vi "Defender.vi"(0 "command\nenum":T13, 2 "Our Robot":T5={"id"=0, "function"=enum."Attacker", "x"=0.0, "y"=0.0, "orientation"=0.0, "v_tangent"=0.0, "v_normal"=0.0, "v_ang"=0.0, "kick_x"=0.0, "kick_z"=0.0, "dribble"=FALSE, "Timestamp"=timestamp(0 s since 1904-01-01), "estimatives"={"est_v_tangent"=0.0, "est_v_normal"=0.0, "est_vx"=0.0, "est_vy"=0.0, "Pos Robot Est"=[]}, "dest_x_kick"=0.0, "dest_y_kick"=0.0, "Gap Coord"=[], "States"=enum."GoToTangent", "Path "=[], "Path  Smooth"=[], "Dest"=[]}, 3 "Atacando contra?":bool=TRUE, 4 "Total de n\natacantes":i32, 5 "Enemy Robots":T5={"id"=0, "function"=enum."Attacker", "x"=0.0, "y"=0.0, "orientation"=0.0, "v_tangent"=0.0, "v_normal"=0.0, "v_ang"=0.0, "kick_x"=0.0, "kick_z"=0.0, "dribble"=FALSE, "Timestamp"=timestamp(0 s since 1904-01-01), "estimatives"={"est_v_tangent"=0.0, "est_v_normal"=0.0, "est_vx"=0.0, "est_vy"=0.0, "Pos Robot Est"=[]}, "dest_x_kick"=0.0, "dest_y_kick"=0.0, "Gap Coord"=[], "States"=enum."GoToTangent", "Path "=[], "Path  Smooth"=[], "Dest"=[]}, 6 "Defensores":u32[](array[numeric]), 7 "geometry":T11, 8 "N atacantes":u32[](array[numeric]), 10 "Total de robos":u32[](array[numeric]), 11 "AI Parameters":T3={"GotoKick"={"Dist do cone a frente"=150.0, "attacker farback"=1500.0, "Perto"=300.0, "min dist to kick"=150.0, "kick eps"=0.0, "Time to transition"=0.05}, "Attacker"={"CC chute"=0.09, "CC passe"=0.045, "Kick Force"=100.0, "ball-robot Kick"=200.0, "ball-robot Pass"=0.3, "drible\nAttk"=FALSE}, "Defender"={"D max"=1700.0, "Vel p/ robô av"=1000.0, "Kick Force"=100.0, "D atk-def"=0.0, "D farback"=0.0, "drible\ndef"=FALSE, "drible\ngoalie"=FALSE}, "Timeout"={"Field/v in x"=6.0, "Dist Robots"=300, "Dist up in y"=300}, "Pose Striker"={"dist"=200.0, "Numeric"=-4.0, "dist 2"=200.0, "drible\nstriker"=FALSE}, "Dist Stop"=300.0, "D ball out"=200, "D central gap "=150.0, "T pass"=0.0, "Force ++"=0.0, "range kick"=0.0, "Chute alto"=TRUE, "Marcador novo"=TRUE, "drible"=FALSE, "D drible"=300.0} {"D drible" format="%#_13g"; "D central gap" format="%#_13g"; "Dist Stop" format="%#_13g"; "Pose Striker"."Numeric" format="%#_13g"; "Defender"."Kick Force" format="%#_13g"; "Defender"."Vel p/ robô av" format="%#_13g"; "Attacker"."ball-robot Kick" format="%#_13g"; "Attacker"."Kick Force" format="%#_13g"; "Attacker"."CC passe" format="%#_13g"; "Attacker"."CC chute" format="%#_13g"; "GotoKick"."kick eps" format="%#_13g"; "GotoKick"."min dist to kick" format="%#_13g"; "GotoKick"."Perto" format="%#_13g"; "GotoKick"."attacker farback" format="%#_13g"; "GotoKick"."Dist do cone a frente" format="%#_13g"}, 12 "total de \ndefensores":i32, 13 "balls":T10[](array[typedef]), 14 "Defesa nova/antiga":T1(ring), 17 "Mais perigoso/segundo mais perigoso":T2(ring)=enum."Marcar o mais perigoso", 18 "IA State Input 2":T4={"our_robots"=[], "enemy_robots"=[], "balls"=[], "geometry"={"line_width"=0, "field_length"=0, "field_width"=0, "boundary_width"=0, "referee_width"=0, "goal_width"=0, "goal_depth"=0, "goal_wall_width"=0, "center_circle_radius"=0, "defense_radius"=0, "defense_stretch"=0, "free_kick_from_defense_dist"=0, "penalty_spot_from_field_line_dist"=0, "penalty_line_from_spot_dist"=0}, "IA Judge"={"stage"="", "command"="", "our_goalie_id"=0.0, "enemy_goalie_id"=0.0, "command enum"=enum."Halt", "Time"=enum."Azul"}, "Received Timestamp"=timestamp(0 s since 1904-01-01), "Events"={"Touch"=FALSE, "Ball out"=FALSE, "id touch"=0.0, "Ball out of \nVision"=FALSE, "Ball inside \nGoalie area"=FALSE, "Robot not responding"=FALSE, "Robots responding status"=[1.0, 1.0, 1.0, 1.0, 1.0, 1.0], "Enemy Ball \nPossession"=FALSE, "Pass State"=FALSE, "id end of pass"=0.0, "Kick"=FALSE, "Id ini Possession"=0.0, "Ball Possesion"=FALSE, "Id Possesion"=0.0}}, 19 "Field defense":dbl[](array[numeric])) -> (15 "output cluster":T5={"id"=0, "function"=enum."Attacker", "x"=0.0, "y"=0.0, "orientation"=0.0, "v_tangent"=0.0, "v_normal"=0.0, "v_ang"=0.0, "kick_x"=0.0, "kick_z"=0.0, "dribble"=FALSE, "Timestamp"=timestamp(0 s since 1904-01-01), "estimatives"={"est_v_tangent"=0.0, "est_v_normal"=0.0, "est_vx"=0.0, "est_vy"=0.0, "Pos Robot Est"=[]}, "dest_x_kick"=0.0, "dest_y_kick"=0.0, "Gap Coord"=[], "States"=enum."GoToTangent", "Path "=[], "Path  Smooth"=[], "Dest"=[]})   [LabVIEW 2017]
uses:
  Core/AI Robot.ctl
  Functions Enum.ctl
  AttackerStates.ctl
  Path Planning/RRT/PathDests.ctl
  Path Planning/RRT/PathDest.ctl
  Command Enum.ctl
  Core/Field Size.ctl
  Core/AI Ball.ctl
  Core/AI Input.ctl
  Core/AI Judge.ctl
  Util/Events/Events.ctl
  AI Parameters.ctl
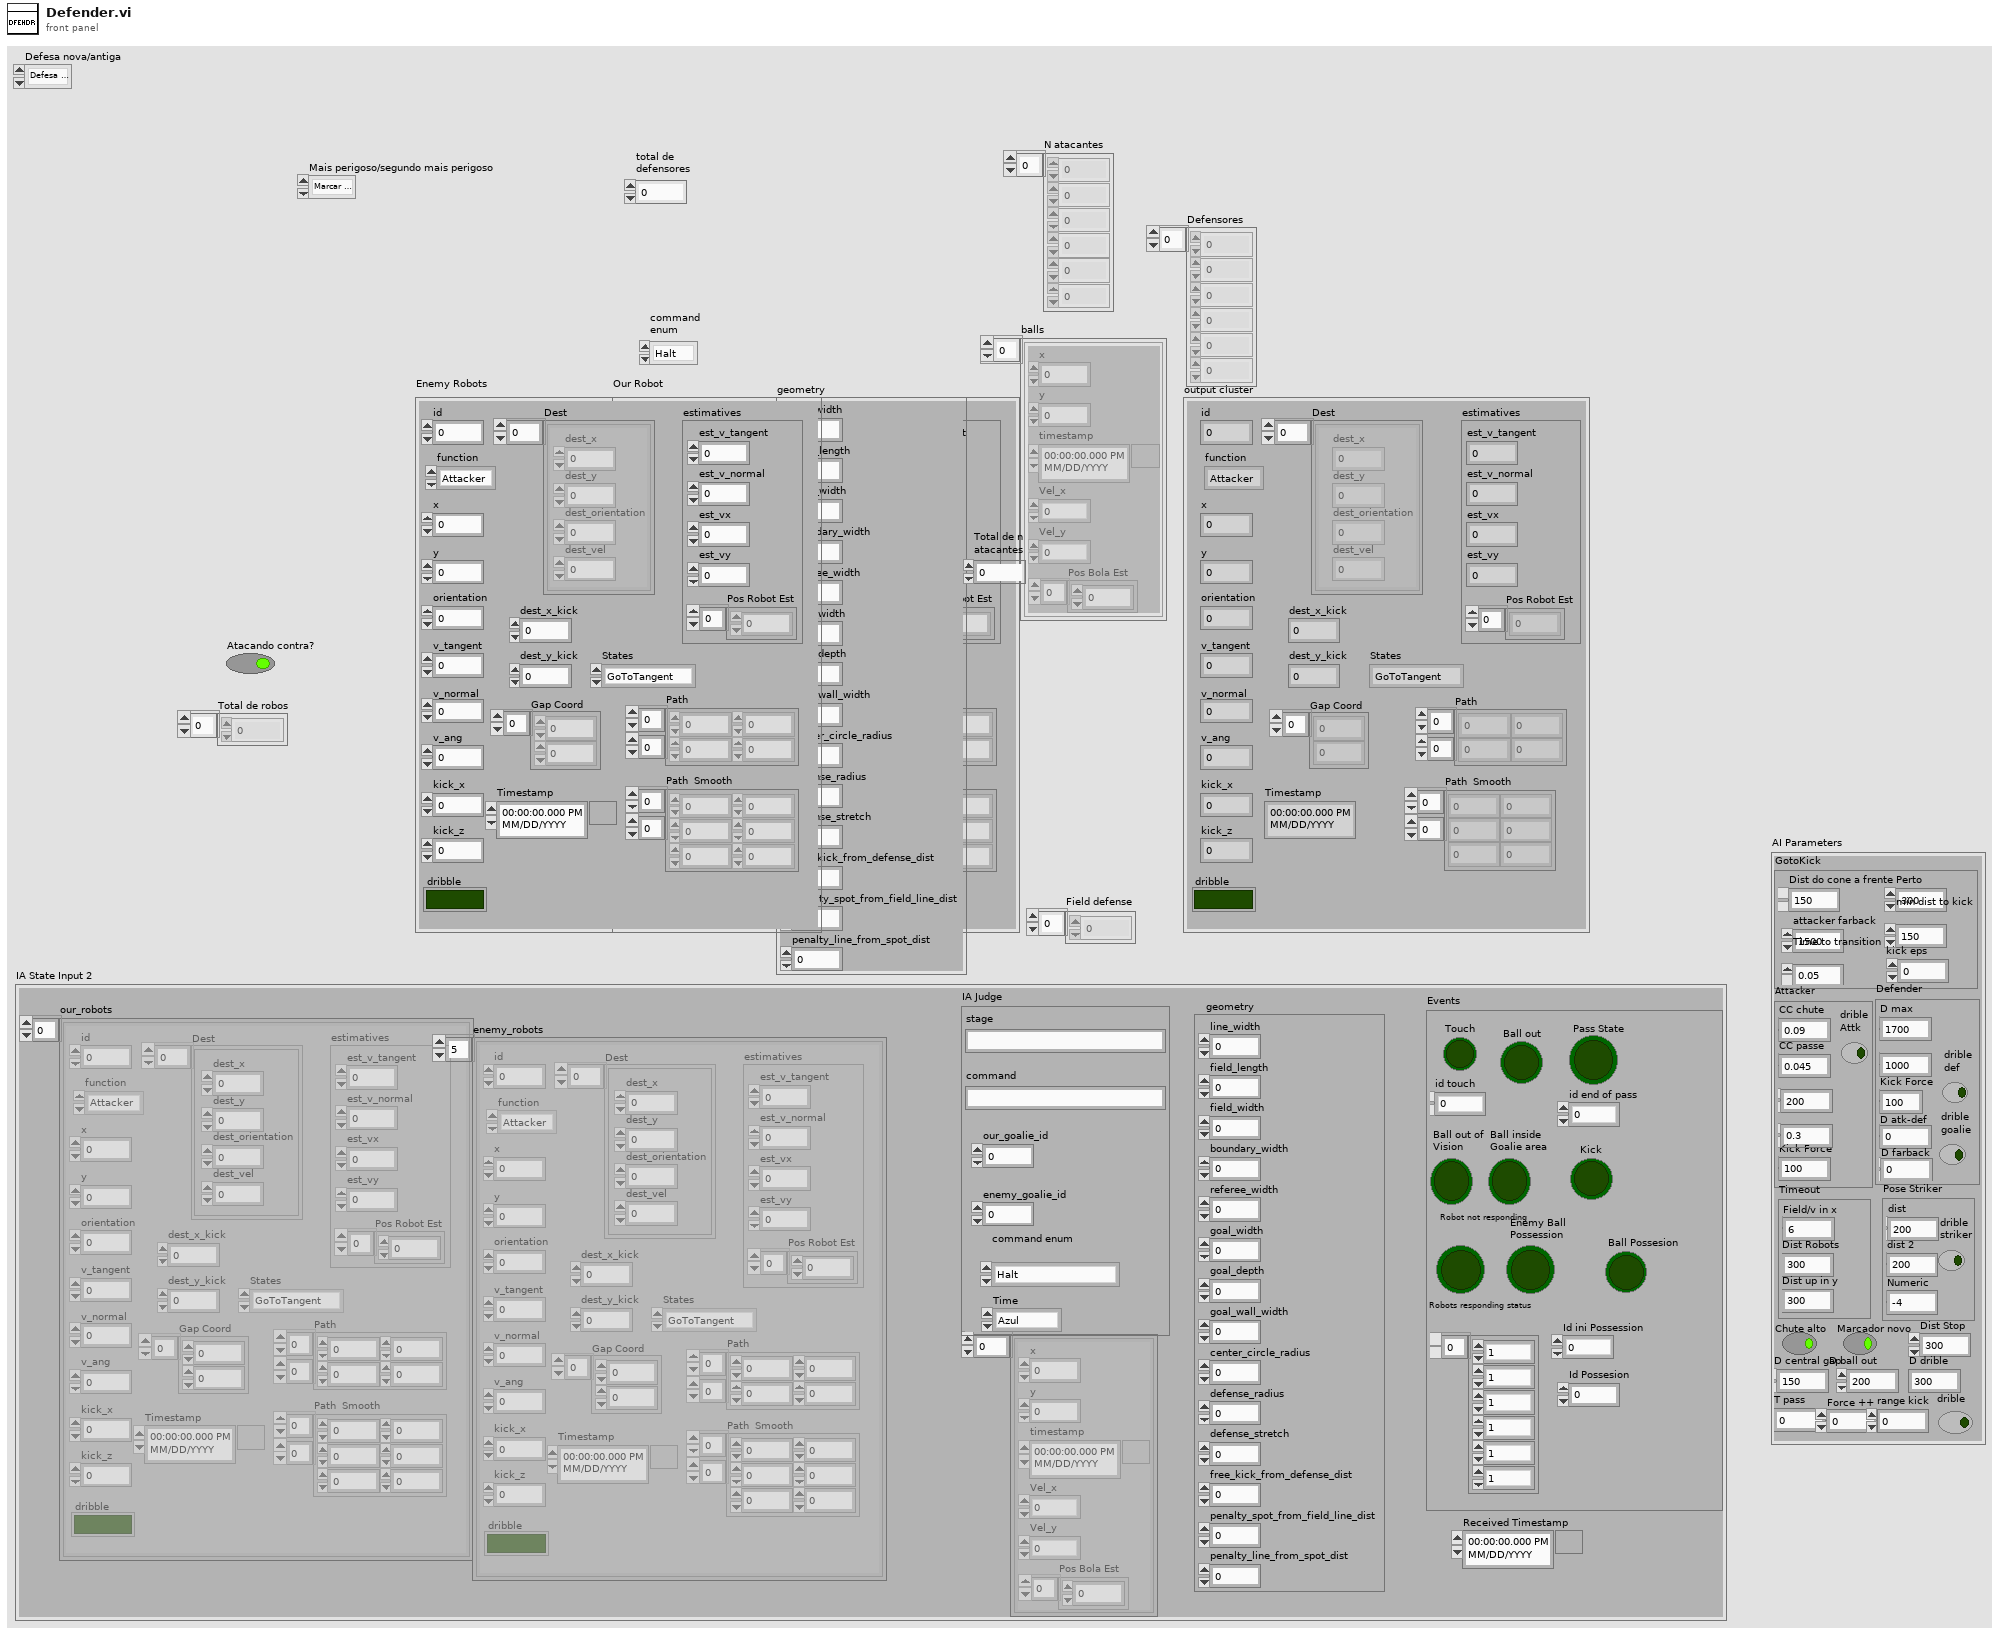
[diagram p1: front panel]
types:
  T1 = enum16{"Defesa Nova(ManMark)", "Defesa Antiga(Barreira)"}
  T2 = enum16{"Marcar Segundo mais perigoso", "Marcar o mais perigoso"}
  T3 = typedef "AI Parameters.ctl" = cluster{"GotoKick":cluster{"Dist do cone a frente":dbl, "attacker farback":dbl, "Perto":dbl, "min dist to kick":dbl, "kick eps":dbl, "Time to transition":dbl}, "Attacker":cluster{"CC chute":dbl, "CC passe":dbl, "Kick Force":dbl, "ball-robot Kick":dbl, "ball-robot Pass":dbl, "drible\nAttk":bool}, "Defender":cluster{"D max":dbl, "Vel p/ robô av":dbl, "Kick Force":dbl, "D atk-def":dbl, "D farback":dbl, "drible\ndef":bool, "drible\ngoalie":bool}, "Timeout":cluster{"Field/v in x":dbl, "Dist Robots":u32, "Dist up in y":u32}, "Pose Striker":cluster{"dist":dbl, "Numeric":dbl, "dist 2":dbl, "drible\nstriker":bool}, "Dist Stop":dbl, "D ball out":i32, "D central gap ":dbl, "T pass":dbl, "Force ++":dbl, "range kick":dbl, "Chute alto":bool, "Marcador novo":bool, "drible":bool, "D drible":dbl}
  T4 = typedef "AI Input.ctl" = cluster{"our_robots":T5[], "enemy_robots":T5[], "balls":T10[], "geometry":T11, "IA Judge":T12, "Received Timestamp":timestamp, "Events":T14}
  T5 = typedef "AI Robot.ctl" = cluster{"id":u32, "function":T6, "x":dbl, "y":dbl, "orientation":dbl, "v_tangent":dbl, "v_normal":dbl, "v_ang":dbl, "kick_x":dbl, "kick_z":dbl, "dribble":bool, "Timestamp":timestamp, "estimatives":cluster{"est_v_tangent":dbl, "est_v_normal":dbl, "est_vx":dbl, "est_vy":dbl, "Pos Robot Est":dbl[]}, "dest_x_kick":dbl, "dest_y_kick":dbl, "Gap Coord":dbl[], "States":T7, "Path ":dbl[][], "Path  Smooth":dbl[][], "Dest":T8}
  T6 = typedef "Functions Enum.ctl" = enum16{"Attacker", "Goalie", "Defender", "Striker", "Goto 0", "Dummy", "Kicker", "ZigZag"}
  T7 = typedef "AttackerStates.ctl" = enum16{"Pass", "GoToTangent", "BallGetting", "GoToKick", ""}
  T8 = typedef "PathDests.ctl" = T9[]
  T9 = typedef "PathDest.ctl" = cluster{"dest_x":dbl, "dest_y":dbl, "dest_orientation":dbl, "dest_vel":dbl}
  T10 = typedef "AI Ball.ctl" = cluster{"x":dbl, "y":dbl, "timestamp":timestamp, "Vel_x":dbl, "Vel_y":dbl, "Pos Bola Est":dbl[]}
  T11 = typedef "Field Size.ctl" = cluster{"line_width":u32, "field_length":u32, "field_width":u32, "boundary_width":u32, "referee_width":u32, "goal_width":u32, "goal_depth":u32, "goal_wall_width":u32, "center_circle_radius":u32, "defense_radius":u32, "defense_stretch":u32, "free_kick_from_defense_dist":u32, "penalty_spot_from_field_line_dist":u32, "penalty_line_from_spot_dist":u32}
  T12 = typedef "AI Judge.ctl" = cluster{"stage":string, "command":string, "our_goalie_id":dbl, "enemy_goalie_id":dbl, "command enum":T13, "Time":enum16{"Azul", "Amarelo"}}
  T13 = typedef "Command Enum.ctl" = enum16{"Halt", "Stop", "Force Start", "PKA Normal Start", "Prepare Kickoff Ally", "PKE Normal Start", "Prepare Kickoff Enemy", "Prepare Penalty Ally", "PPA Normal Start", "Prepare Penalty Enemy", "PPE Normal Start", "Direct Free Enemy", "Direct Free Ally", "Indirect Free Enemy", "Indirect Free Ally", "Timeout Enemy", "Timeout Ally", "Goal Enemy", "Goal Ally", "Ball Placement Enemy", "Ball Placement Ally", "Normal Half Time", "Extra Time Break", "Extra Half Time", "None", "Post Game"}
  T14 = typedef "Events.ctl" = cluster{"Touch":bool, "Ball out":bool, "id touch":dbl, "Ball out of \nVision":bool, "Ball inside \nGoalie area":bool, "Robot not responding":bool, "Robots responding status":dbl[], "Enemy Ball \nPossession":bool, "Pass State":bool, "id end of pass":dbl, "Kick":bool, "Id ini Possession":dbl, "Ball Possesion":bool, "Id Possesion":dbl}
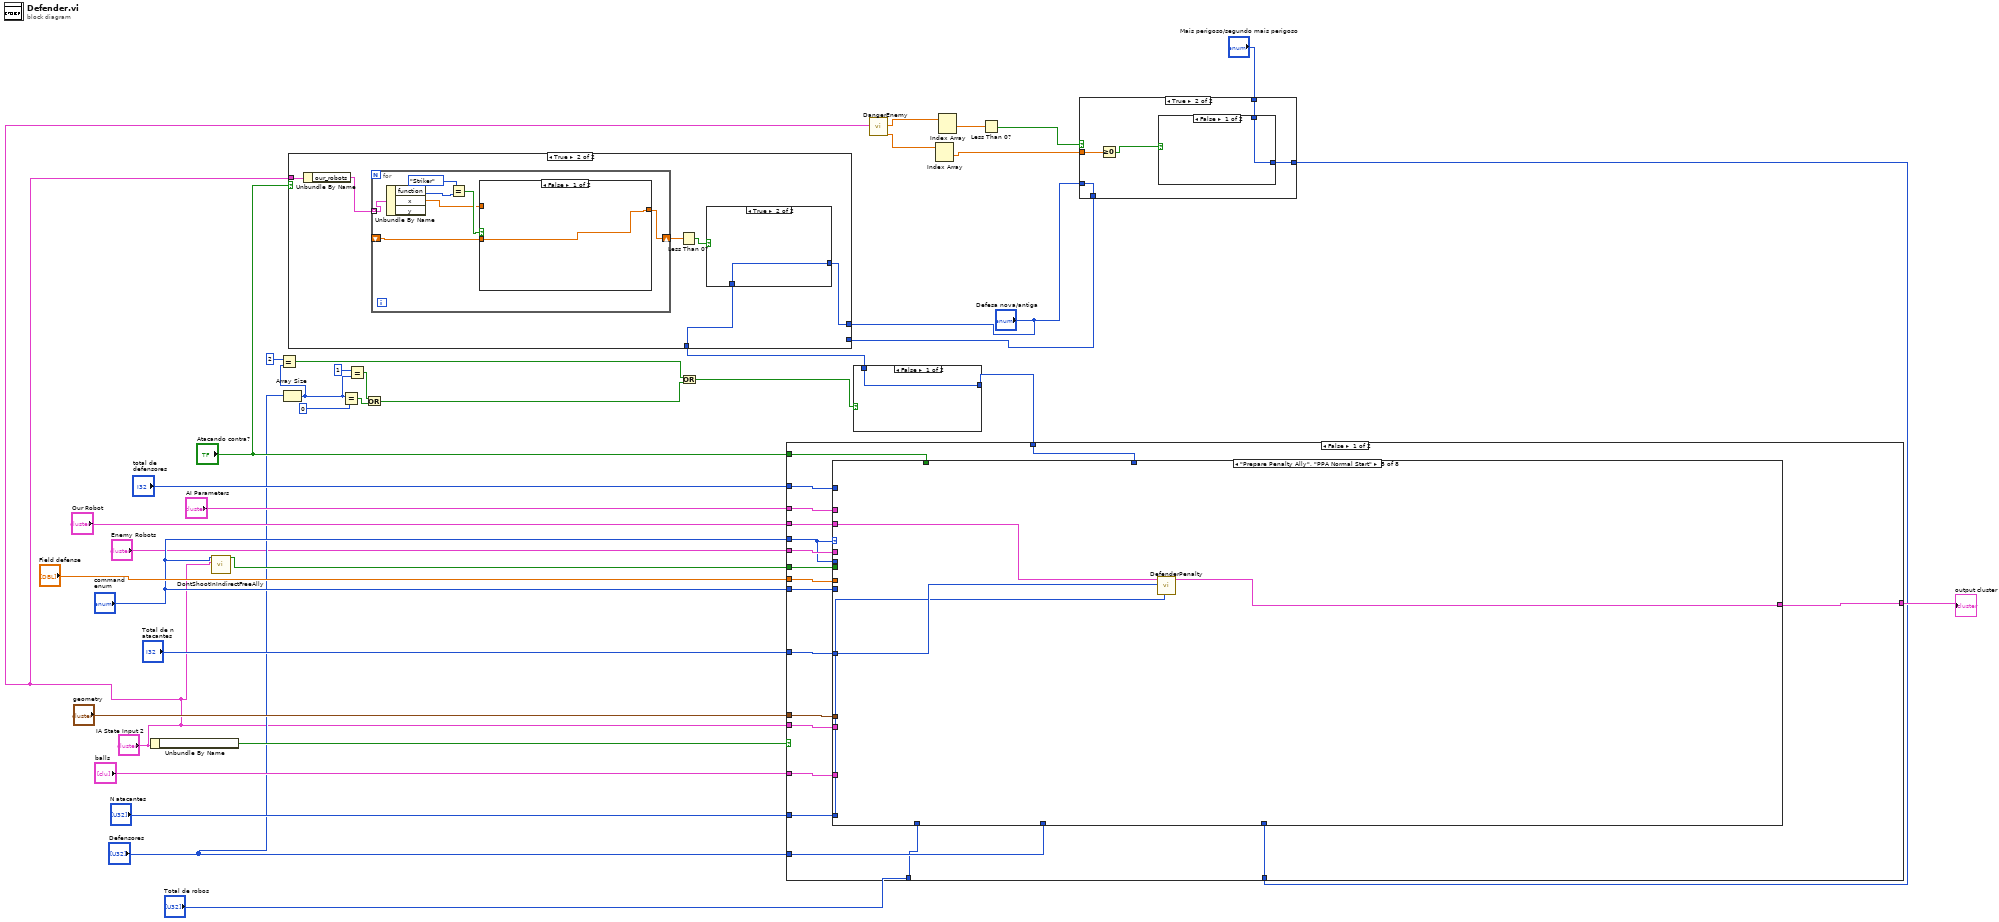
[diagram p0: block diagram]
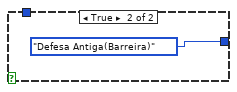
[diagram p2: hidden frame]
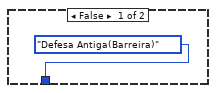
[diagram p4: hidden frame]
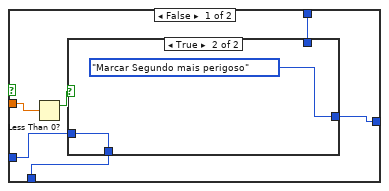
[diagram p6: hidden frame]
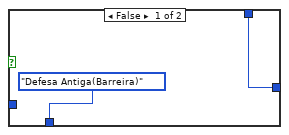
[diagram p7: hidden frame]
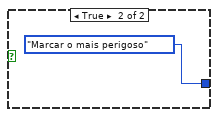
[diagram p8: hidden frame]
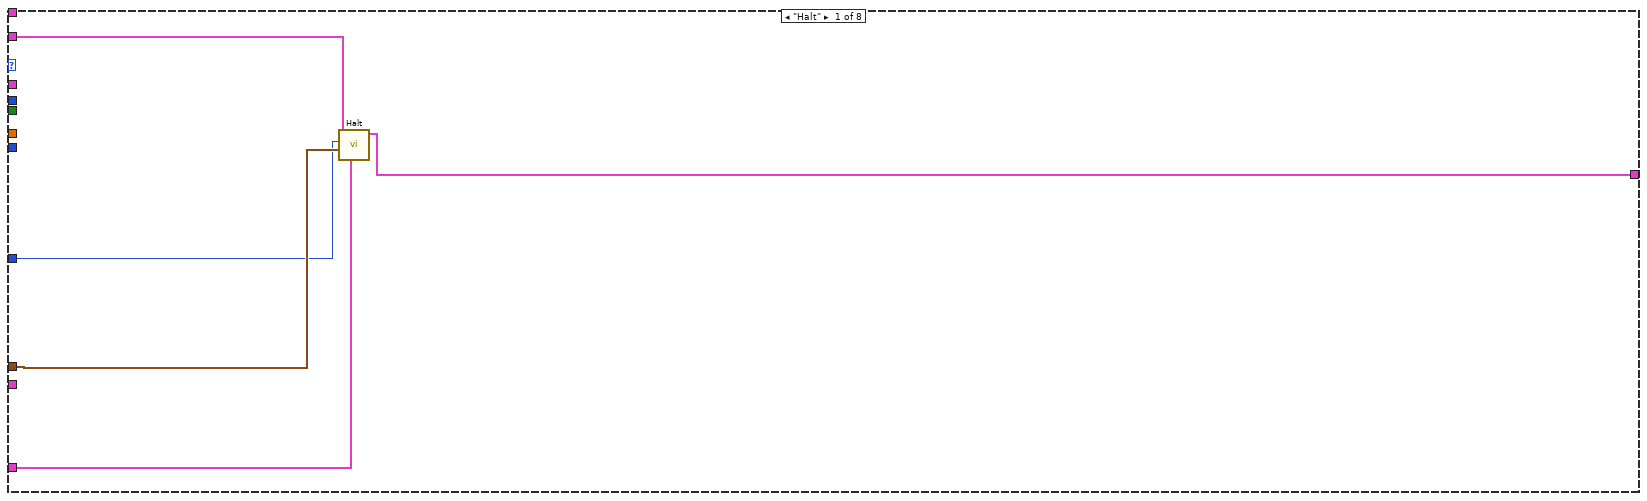
[diagram p9: hidden frame]
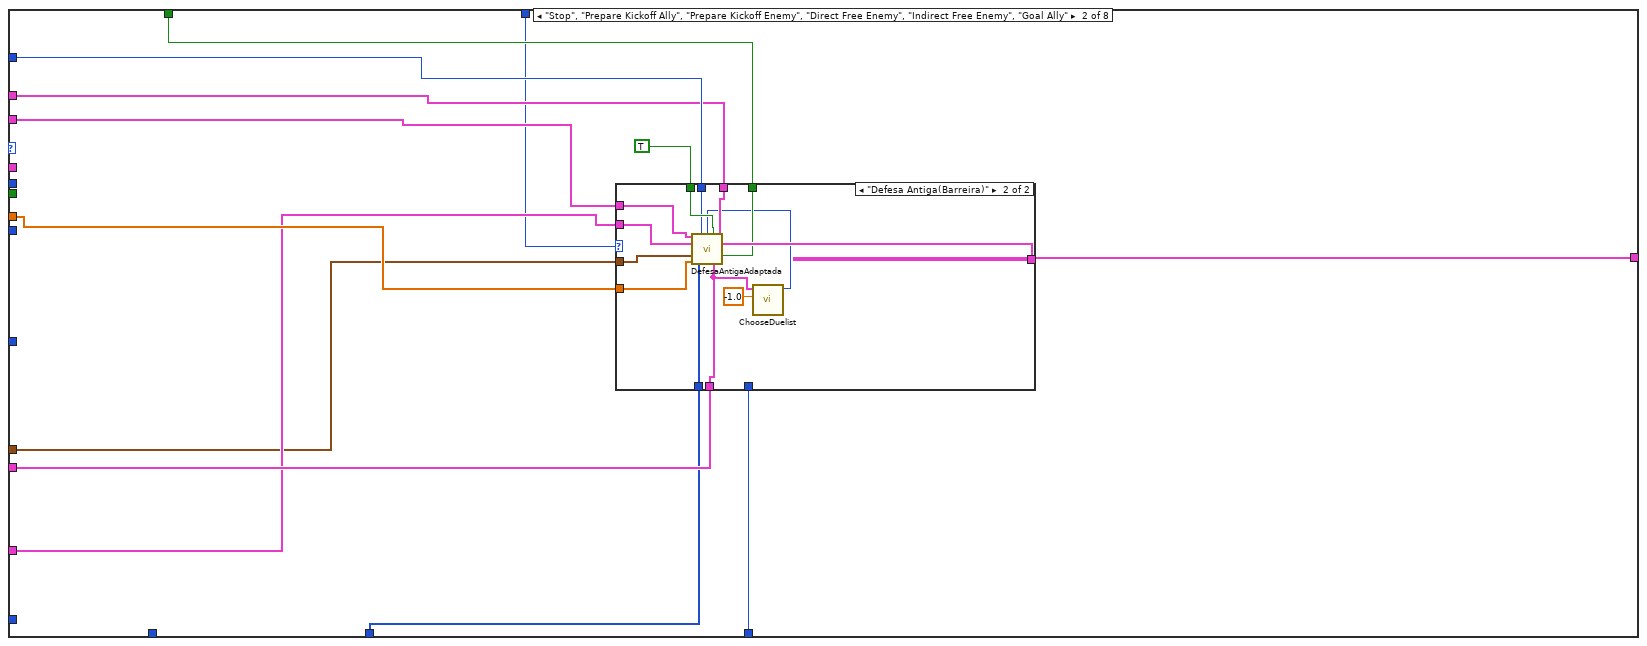
[diagram p10: hidden frame]
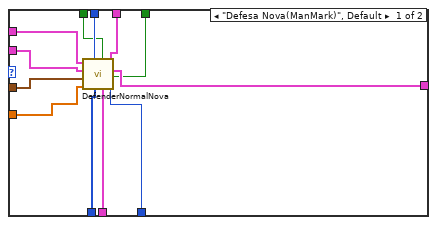
[diagram p11: hidden frame]
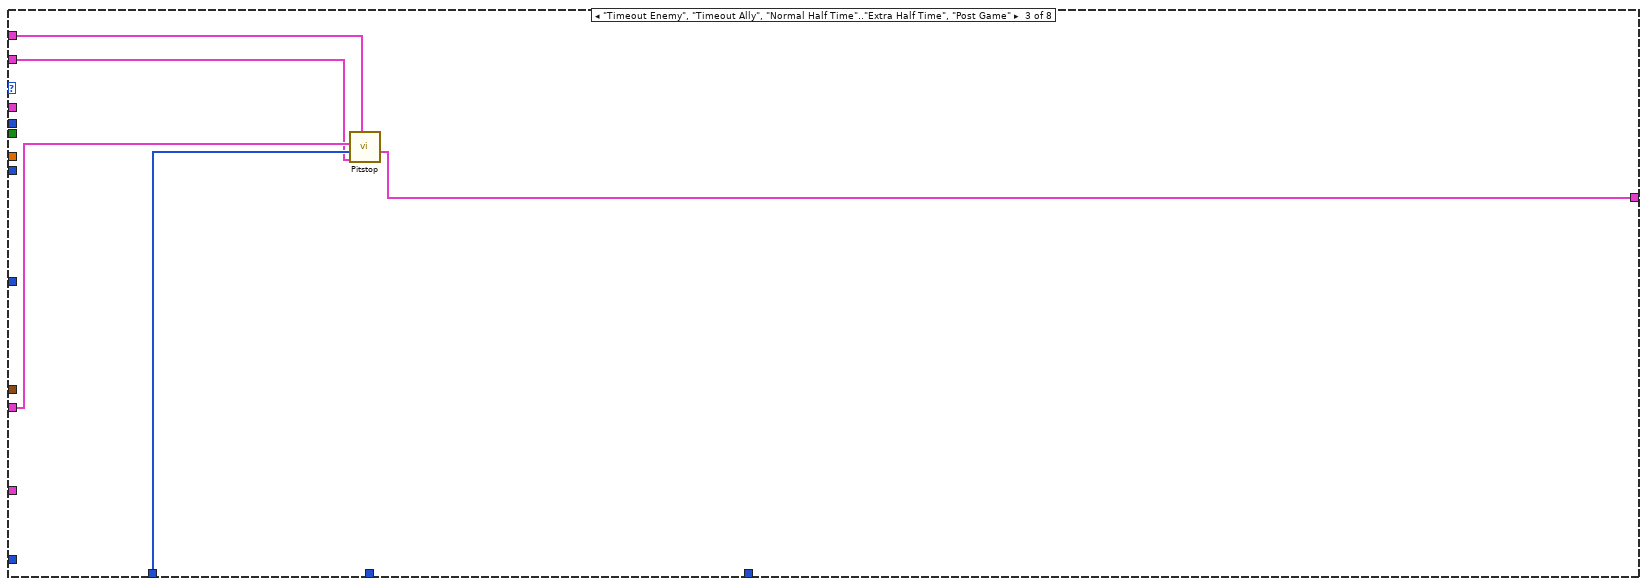
[diagram p12: hidden frame]
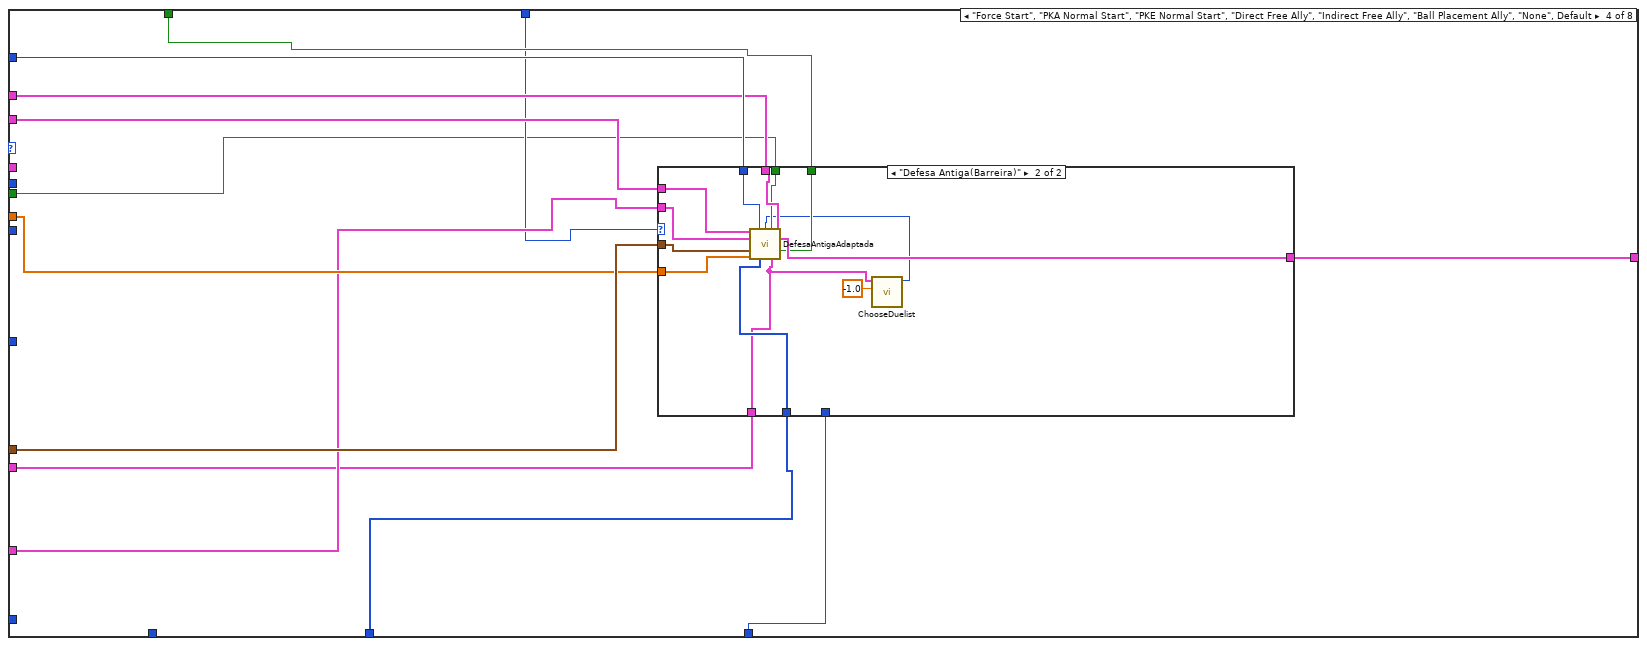
[diagram p13: hidden frame]
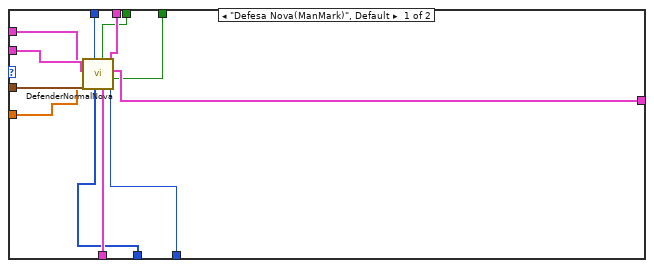
[diagram p14: hidden frame]
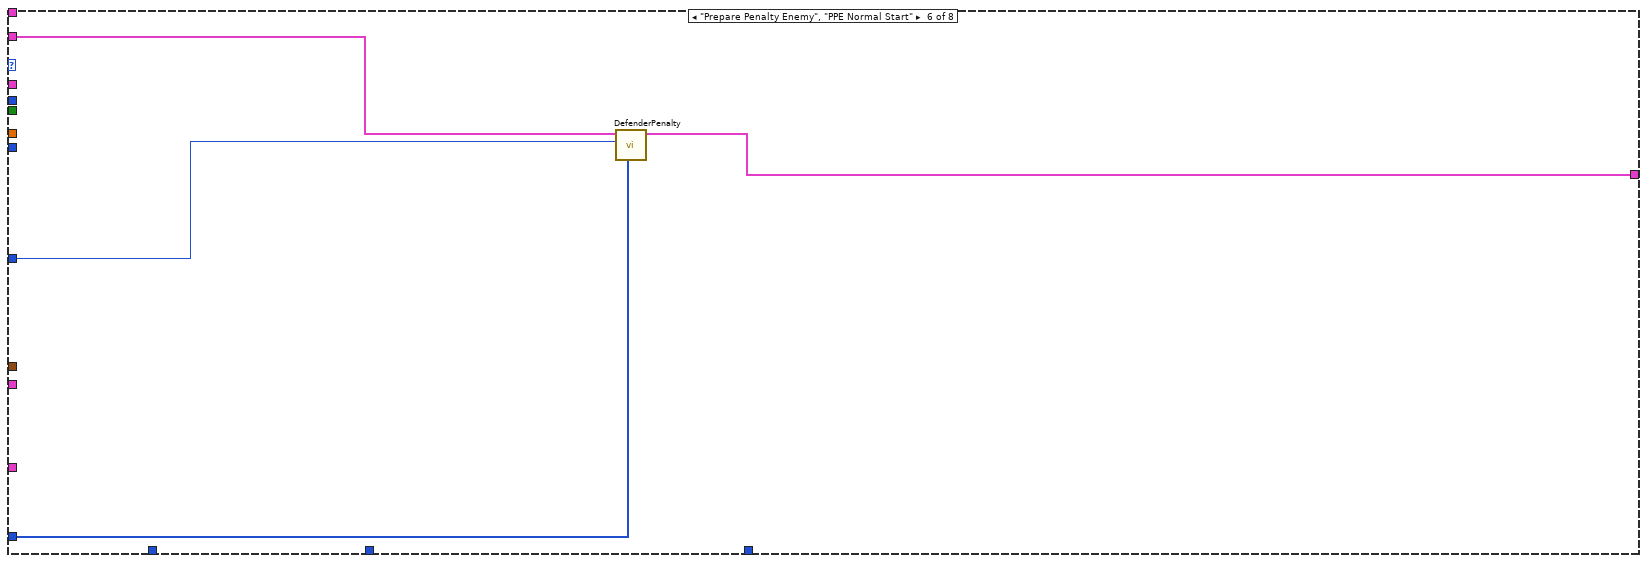
[diagram p15: hidden frame]
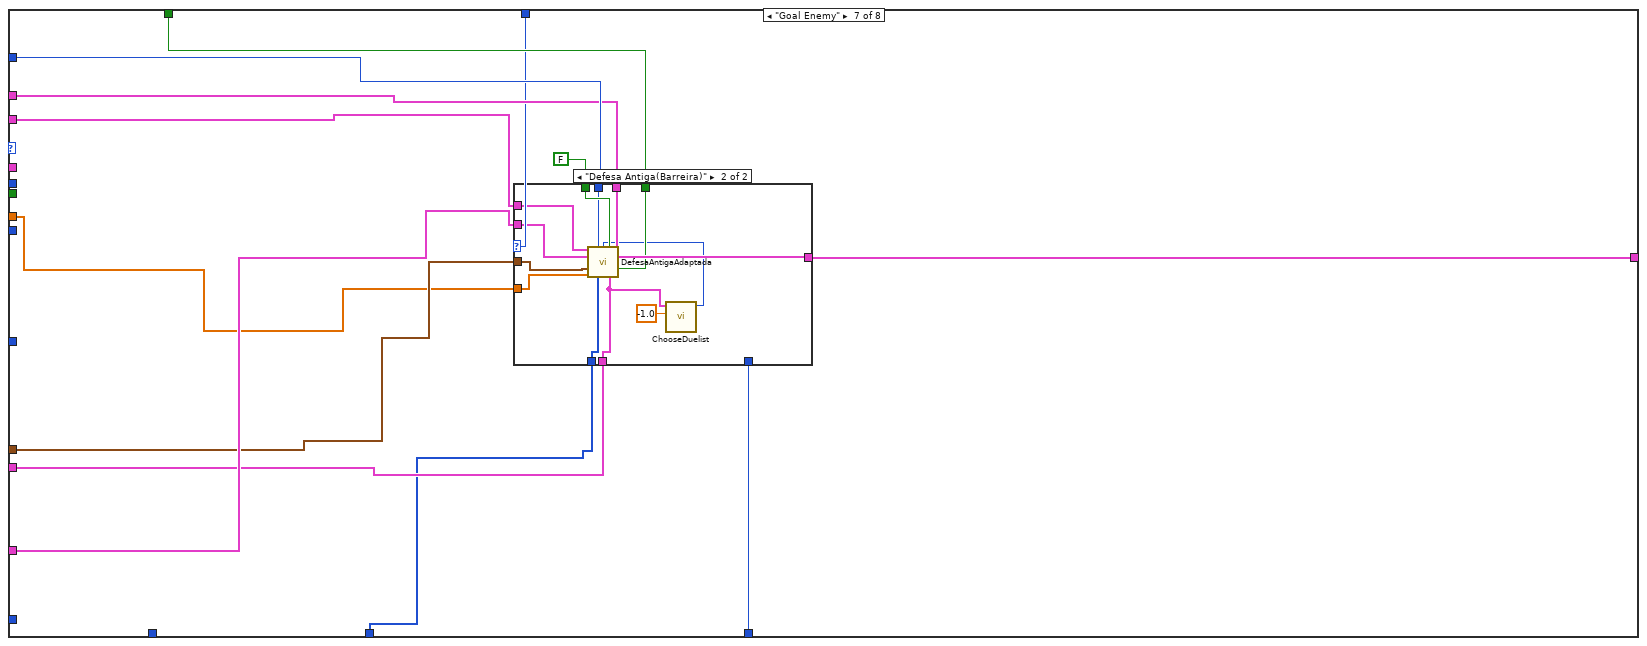
[diagram p16: hidden frame]
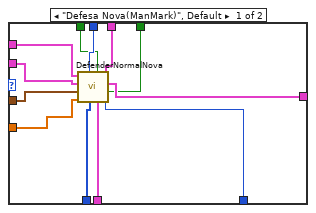
[diagram p17: hidden frame]
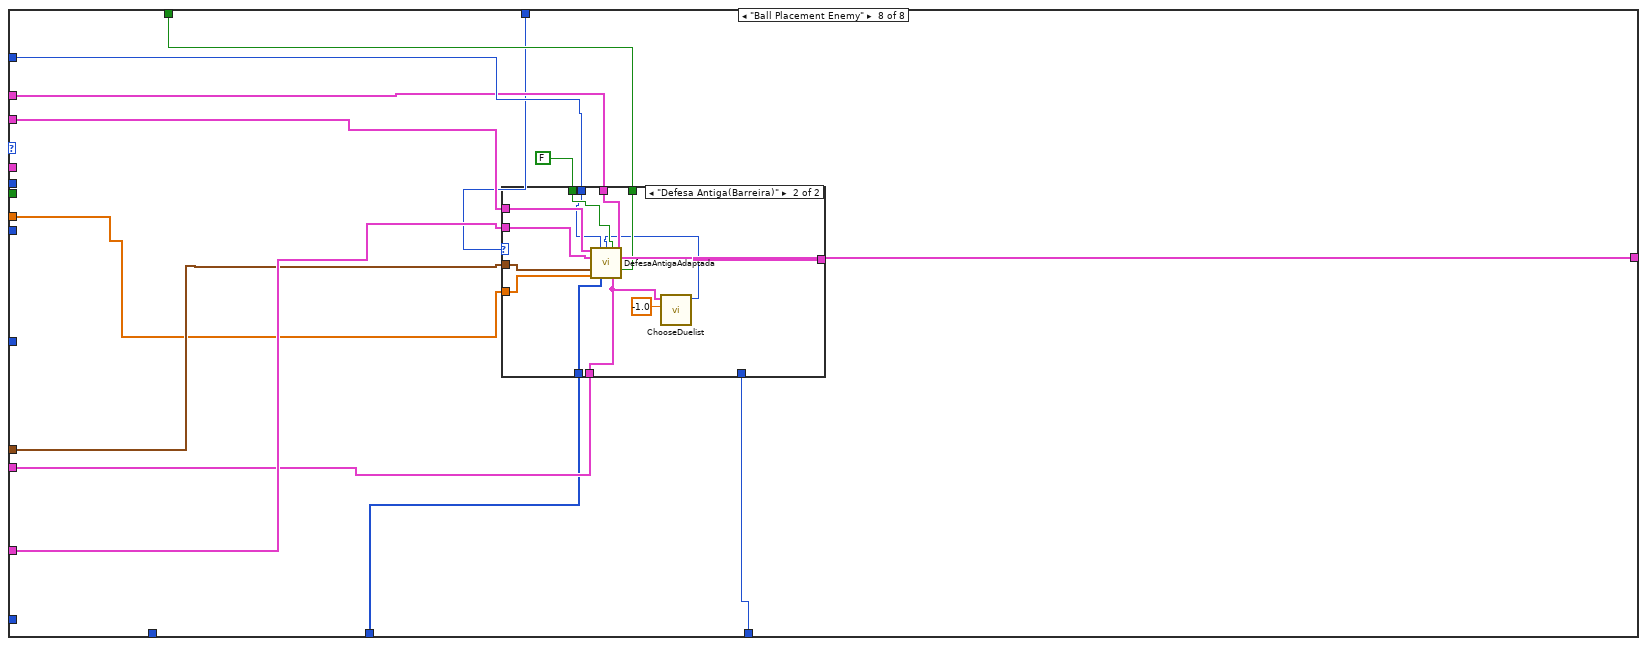
[diagram p18: hidden frame]
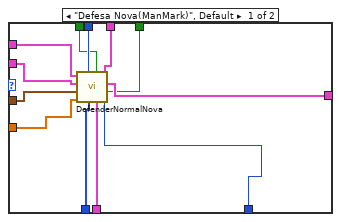
[diagram p19: hidden frame]
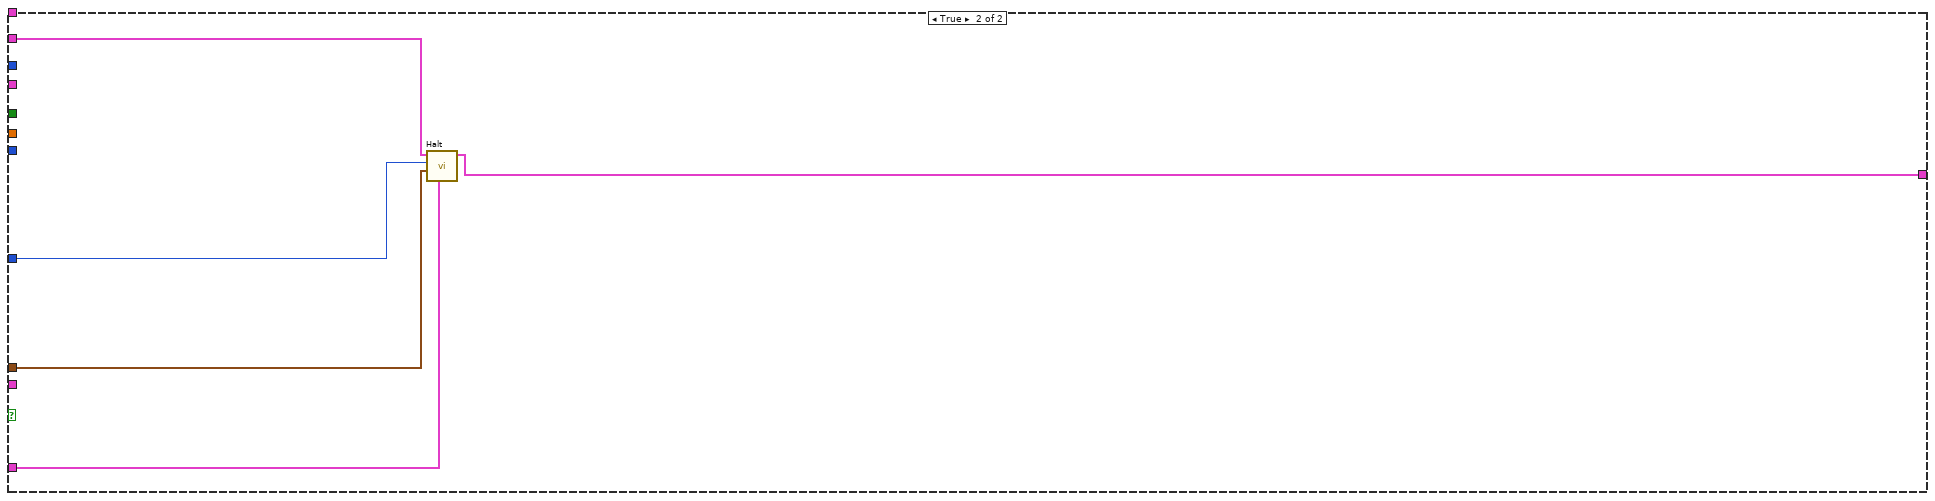
[diagram p20: hidden frame]
diagram:
  n1 = Unbundle By Name("IA State Input 2") -> ("Events.Ball out of \nVision"=w29:bool)
  n2 = call "DontShootInIndirectFreeAlly.vi"("IA State Input 2"="IA State Input 2", "command\nenum"="command\nenum") -> ("Stop?"=w15:bool)  [unwired: 9 in]
  n3 = Array Size(array="Defensores") -> (size(s)=w6:i32)
  n4 = Equal?(x=2, y=w6) -> (x = y?=w4:bool)
  n5 = Equal?(x=w6, y=0) -> (x = y?=w11:bool)
  n6 = Equal?(x=1, y=w6) -> (x = y?=w10:bool)
  n7 = Or(x=w10, y=w11) -> (x .or. y?=w7:bool)
  n8 = Or(x=w4, y=w7) -> (x .or. y?=w3:bool)
  n9 = call "DangerEnemy.vi"("IA Input"="IA State Input 2") -> ("Pos do segundo inimigo\nperigoso"=w23:dbl[], "Pos do inimigo\nperigoso"=w26:dbl[])  [unwired: 7 in, 2 out]
  n10 = Index Array(array=w23) -> (element #1=w22:dbl)  [unwired: 2 in, 1 out]
  n11 = Index Array(array=w26) -> (element #1=w25:dbl)  [unwired: 2 in, 1 out]
  n12 = Less Than 0?(x=w25) -> (x < 0?=w24:bool)
  n13 = case shown="True" w24 {
    tunnel: [w41 w52] -> w18
    tunnel: "Defesa nova/antiga" -> [w38 w52]
    tunnel: w22 -> [w43 w51]
    tunnel: [w40 w49] -> w17
    tunnel: "Mais perigoso/segundo mais perigoso" -> [w39 w48]
    frame False {
      n14 = Less Than 0?(x=w43) -> (x < 0?=w42:bool)
      n15 = case shown="True" w42 {
        tunnel: [T1."Defesa Antiga(Barreira)" ("Defesa nova/antiga") w46] -> w41
        tunnel: [w44 T2."Marcar Segundo mais perigoso" ("Mais perigoso/segundo mais perigoso 2")] -> w40
        tunnel: w39 -> [w44 _]
        tunnel: w38 -> [_ w46]
        frame False {
        }
        frame True {
        }
      }
    }
    frame True {
      n16 = Greater Or Equal To 0?(x=w51) -> (x >= 0?=w50:bool)
      n17 = case shown="False" w50 {
        tunnel: [w53 T2."Marcar o mais perigoso" ("Mais perigoso/segundo mais perigoso 2")] -> w49
        tunnel: w48 -> [w53 _]
        frame False {
        }
        frame True {
        }
      }
    }
  }
  n18 = case shown="True" "Atacando contra?" {
    tunnel: [w55 w57] -> w8
    tunnel: "Defesa nova/antiga" -> [_ w56]
    tunnel: w18 -> [w55 _]
    tunnel: "IA State Input 2" -> [_ w61]
    frame False {
    }
    frame True {
      n19 = Unbundle By Name(w61) -> ("our_robots"=w60:T5[])
      n20 = for {
        tunnel: w60 -> [w70] mode=indexing
        shift-right: [w66] -> w59
        shift-left: _ -> [w64]
        n21 = Unbundle By Name(w70) -> ("function"=w69:T6, "x"=w65:dbl)  [unwired: 1 out]
        n22 = Equal?(x=Functions_Enum."Striker", y=w69) -> (x = y?=w67:bool)
        n23 = case shown="False" w67 {
          tunnel: [w71 w72] -> w66
          tunnel: w65 -> [_ w72]
          tunnel: w64 -> [w71 _]
          frame False {
          }
          frame True {
          }
        }
      }
      n24 = Less Than 0?(x=w59) -> (x < 0?=w58:bool)
      n25 = case shown="True" w58 {
        tunnel: [T1."Defesa Antiga(Barreira)" ("Defesa nova/antiga") w63] -> w57
        tunnel: w56 -> [_ w63]
        frame False {
        }
        frame True {
        }
      }
    }
  }
  n26 = case shown="False" w3 {
    tunnel: [w73 T1."Defesa Antiga(Barreira)" ("Defesa nova/antiga")] -> w9
    tunnel: w8 -> [w73 _]
    frame False {
    }
    frame True {
    }
  }
  n27 = case shown="False" w29 {
    tunnel: [w93 w264] -> w37
    tunnel: "Our Robot" -> [w92 w268]
    tunnel: "command\nenum" -> [w82 _]
    tunnel: "balls" -> [w91 w265]
    tunnel: "geometry" -> [w90 w266]
    tunnel: "Total de n\natacantes" -> [w89 w267]
    tunnel: "total de \ndefensores" -> [w88 _]
    tunnel: "Enemy Robots" -> [w87 _]
    tunnel: "Defensores" -> [w86 _]
    tunnel: "N atacantes" -> [w85 _]
    tunnel: "Field defense" -> [w84 _]
    tunnel: "IA State Input 2" -> [w83 _]
    tunnel: "Total de robos" -> [w81 _]
    tunnel: "AI Parameters" -> [w80 _]
    tunnel: "Atacando contra?" -> [w79 _]
    tunnel: w9 -> [w78 _]
    tunnel: w17 -> [w77 _]
    tunnel: "command\nenum" -> [w76 _]
    tunnel: w15 -> [w75 _]
    frame False {
      n28 = case shown="\"Prepare Penalty Ally\", \"PPA Normal Start\"" w82 {
        tunnel: w92 -> [w94 w102 w138 w148 w183 w187 w192 w234]
        tunnel: [w98 w111 w139 w154 w181 w185 w191 w229] -> w93
        tunnel: w91 -> [w97 w107 _ w149 _ _ w196 w233]
        tunnel: w90 -> [w96 w106 _ w151 _ _ w194 w232]
        tunnel: w89 -> [w95 _ _ _ w182 w186 _ _]
        tunnel: w88 -> [_ w105 _ w153 _ _ w200 w237]
        tunnel: w87 -> [_ _ _ _ _ _ _ _]
        tunnel: w86 -> [_ w109 _ w146 _ _ w190 w228]
        tunnel: w85 -> [_ _ _ _ w180 w184 _ _]
        tunnel: w84 -> [_ w108 _ w150 _ _ w193 w231]
        tunnel: w83 -> [_ w110 w141 w143 _ _ w195 w230]
        tunnel: w82 -> [_ _ _ _ _ _ _ _]
        tunnel: w81 -> [_ _ w140 _ _ _ _ _]
        tunnel: w80 -> [_ w103 w137 w147 _ _ w199 w235]
        tunnel: w79 -> [_ w104 _ w152 _ _ w198 w236]
        tunnel: w78 -> [_ w100 _ w145 _ _ w189 w227]
        tunnel: w77 -> [_ w99 _ w144 _ _ w188 w226]
        tunnel: w76 -> [_ _ _ _ _ _ _ _]
        tunnel: w75 -> [_ _ _ w142 _ _ _ _]
        frame "Halt" {
          n29 = call "Halt.vi"("balls"=w97, "Field Size in"=w96, "Numeric"=w95, "Robot in"=w94) -> ("Robot out"=w98:T5)  [unwired: 7 in]
        }
        frame "Stop", "Prepare Kickoff Ally", "Prepare Kickoff Enemy", "Direct Free Enemy", "Indirect Free Enemy", "Goal Ally" {
          n30 = case shown="\"Defesa Antiga(Barreira)\"" w100 {
            tunnel: [w123 w136] -> w111
            tunnel: w105 -> [w122 w128]
            tunnel: w104 -> [w121 w129]
            tunnel: w110 -> [w120 w125]
            tunnel: w109 -> [w119 w127]
            tunnel: w106 -> [w112 w131]
            tunnel: w108 -> [w118 w130]
            tunnel: w107 -> [w117 w132]
            tunnel: w102 -> [w116 w133]
            tunnel: w103 -> [w115 w134]
            tunnel: TRUE ("Stop?") -> [w114 w135]
            tunnel: w99 -> [w113 _]
            frame "Defesa Nova(ManMark)", Default {
              n31 = call "DefenderNormalNova.vi"("Enum"=w113, "Atacando contra?"=w121, "AI Parameters"=w115, "IA State Input 2"=w120, "Stop?"=w114, "Defensores"=w119, "total de \ndefensores"=w122, "Field defense"=w118, "geometry"=w112, "balls"=w117, "Our Robot"=w116) -> ("Robot out"=w123:T5)
            }
            frame "Defesa Antiga(Barreira)" {
              n32 = call "ChooseDuelist.vi"("Id Manmarker"=-1.0, "IA State Input 2"=w125) -> ("Id Duelist"=w124:u32)  [unwired: 8 in, 1 out]
              n33 = call "DefesaAntigaAdaptada.vi"("Our Robot"=w133, "total de \ndefensores"=w128, "Id duelist"=w124, "Stop?"=w135, "AI Parameters"=w134, "balls"=w132, "Field Size 2"=w131, "Atacando contra?"=w129, "Field defense"=w130, "Defensores"=w127, "IA State Input 2"=w125) -> ("Robot out"=w136:T5)  [unwired: 4 in]
            }
          }
        }
        frame "Timeout Enemy", "Timeout Ally", "Normal Half Time".."Extra Half Time", "Post Game" {
          n34 = call "Pitstop.vi"("AI Parameters"=w137, "Robot in"=w138, "robos"=w140, "IA State Input"=w141) -> ("Robot out"=w139:T5)  [unwired: 7 in]
        }
        frame "Force Start", "PKA Normal Start", "PKE Normal Start", "Direct Free Ally", "Indirect Free Ally", "Ball Placement Ally", "None", Default {
          n35 = case shown="\"Defesa Antiga(Barreira)\"" w145 {
            tunnel: [w166 w179] -> w154
            tunnel: w153 -> [w165 w172]
            tunnel: w152 -> [w164 w174]
            tunnel: w143 -> [w163 w168]
            tunnel: w151 -> [w162 w178]
            tunnel: w150 -> [w161 w177]
            tunnel: w149 -> [w160 w176]
            tunnel: w148 -> [w159 w175]
            tunnel: w147 -> [w158 w173]
            tunnel: w146 -> [w157 w170]
            tunnel: w144 -> [w156 _]
            tunnel: w142 -> [w155 w171]
            frame "Defesa Nova(ManMark)", Default {
              n36 = call "DefenderNormalNova.vi"("Enum"=w156, "Atacando contra?"=w164, "AI Parameters"=w158, "IA State Input 2"=w163, "Stop?"=w155, "Defensores"=w157, "total de \ndefensores"=w165, "Field defense"=w161, "geometry"=w162, "balls"=w160, "Our Robot"=w159) -> ("Robot out"=w166:T5)
            }
            frame "Defesa Antiga(Barreira)" {
              n37 = call "ChooseDuelist.vi"("Id Manmarker"=-1.0, "IA State Input 2"=w168) -> ("Id Duelist"=w167:u32)  [unwired: 8 in, 1 out]
              n38 = call "DefesaAntigaAdaptada.vi"("Our Robot"=w175, "total de \ndefensores"=w172, "Id duelist"=w167, "Stop?"=w171, "AI Parameters"=w173, "balls"=w176, "Field Size 2"=w178, "Atacando contra?"=w174, "Field defense"=w177, "Defensores"=w170, "IA State Input 2"=w168) -> ("Robot out"=w179:T5)  [unwired: 4 in]
            }
          }
        }
        frame "Prepare Penalty Ally", "PPA Normal Start" {
          n39 = call "DefenderPenalty.vi"("N atacantes"=w180, "Total de n \natacantes"=w182, "Robot in"=w183) -> ("Robot out"=w181:T5)  [unwired: 8 in]
        }
        frame "Prepare Penalty Enemy", "PPE Normal Start" {
          n40 = call "DefenderPenalty.vi"("N atacantes"=w184, "Total de n \natacantes"=w186, "Robot in"=w187) -> ("Robot out"=w185:T5)  [unwired: 8 in]
        }
        frame "Goal Enemy" {
          n41 = case shown="\"Defesa Antiga(Barreira)\"" w189 {
            tunnel: [w212 w225] -> w191
            tunnel: w200 -> [w211 w222]
            tunnel: w198 -> [w210 w223]
            tunnel: w195 -> [w209 w214]
            tunnel: w190 -> [w208 w216]
            tunnel: w194 -> [w207 w219]
            tunnel: w193 -> [w206 w218]
            tunnel: w196 -> [w205 w220]
            tunnel: w192 -> [w204 w221]
            tunnel: w199 -> [w203 w217]
            tunnel: FALSE ("Stop?") -> [w202 w224]
            tunnel: w188 -> [w201 _]
            frame "Defesa Nova(ManMark)", Default {
              n42 = call "DefenderNormalNova.vi"("Enum"=w201, "Atacando contra?"=w210, "AI Parameters"=w203, "IA State Input 2"=w209, "Stop?"=w202, "Defensores"=w208, "total de \ndefensores"=w211, "Field defense"=w206, "geometry"=w207, "balls"=w205, "Our Robot"=w204) -> ("Robot out"=w212:T5)
            }
            frame "Defesa Antiga(Barreira)" {
              n43 = call "ChooseDuelist.vi"("Id Manmarker"=-1.0, "IA State Input 2"=w214) -> ("Id Duelist"=w213:u32)  [unwired: 8 in, 1 out]
              n44 = call "DefesaAntigaAdaptada.vi"("Our Robot"=w221, "total de \ndefensores"=w222, "Id duelist"=w213, "Stop?"=w224, "AI Parameters"=w217, "balls"=w220, "Field Size 2"=w219, "Atacando contra?"=w223, "Field defense"=w218, "Defensores"=w216, "IA State Input 2"=w214) -> ("Robot out"=w225:T5)  [unwired: 4 in]
            }
          }
        }
        frame "Ball Placement Enemy" {
          n45 = case shown="\"Defesa Antiga(Barreira)\"" w227 {
            tunnel: [w250 w263] -> w229
            tunnel: w237 -> [w249 w257]
            tunnel: w236 -> [w248 w261]
            tunnel: w230 -> [w247 w252]
            tunnel: w228 -> [w246 w254]
            tunnel: w232 -> [w245 w256]
            tunnel: w231 -> [w244 w255]
            tunnel: w233 -> [w243 w259]
            tunnel: w234 -> [w242 w260]
            tunnel: w235 -> [w241 w262]
            tunnel: FALSE ("Stop?") -> [w240 w258]
            tunnel: w226 -> [w239 _]
            frame "Defesa Nova(ManMark)", Default {
              n46 = call "DefenderNormalNova.vi"("Enum"=w239, "Atacando contra?"=w248, "AI Parameters"=w241, "IA State Input 2"=w247, "Stop?"=w240, "Defensores"=w246, "total de \ndefensores"=w249, "Field defense"=w244, "geometry"=w245, "balls"=w243, "Our Robot"=w242) -> ("Robot out"=w250:T5)
            }
            frame "Defesa Antiga(Barreira)" {
              n47 = call "ChooseDuelist.vi"("Id Manmarker"=-1.0, "IA State Input 2"=w252) -> ("Id Duelist"=w251:u32)  [unwired: 8 in, 1 out]
              n48 = call "DefesaAntigaAdaptada.vi"("Our Robot"=w260, "total de \ndefensores"=w257, "Id duelist"=w251, "Stop?"=w258, "AI Parameters"=w262, "balls"=w259, "Field Size 2"=w256, "Atacando contra?"=w261, "Field defense"=w255, "Defensores"=w254, "IA State Input 2"=w252) -> ("Robot out"=w263:T5)  [unwired: 4 in]
            }
          }
        }
      }
    }
    frame True {
      n49 = call "Halt.vi"("balls"=w265, "Field Size in"=w266, "Numeric"=w267, "Robot in"=w268) -> ("Robot out"=w264:T5)  [unwired: 7 in]
    }
  }
  "output cluster" <- w37
